vi "Grid_Read Control.vi"(8 "error in (no error)":errorcluster, 11 "Grid in":refnum<class "Grid.lvclass">) -> (0 "error out":errorcluster, 2 "Control":T1, 3 "Grid out":refnum<class "Grid.lvclass">)   [LabVIEW 2015, in "Grid.lvclass"]
uses:
  Grid.lvclass
  Grid_Control.ctl
  Grid.lvclass/Grid.ctl
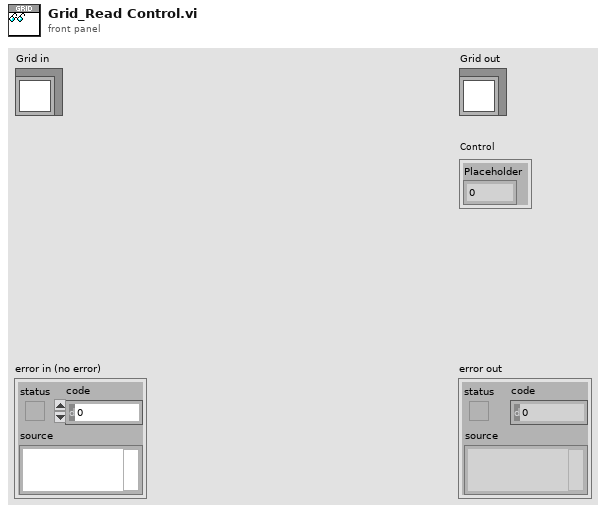
[diagram p1: front panel]
types:
  T1 = typedef "Grid.lvclass/Grid_Control.ctl" = cluster{"Placeholder":dbl}
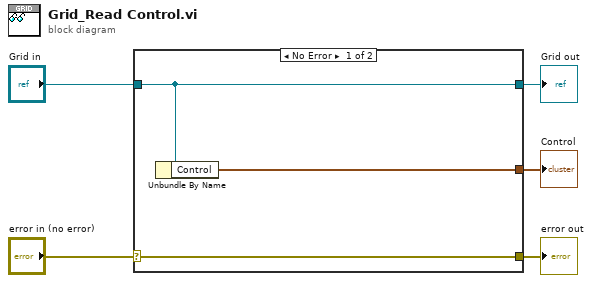
[diagram p0: block diagram]
diagram:
  n1 = case shown="No Error" "error in (no error)" {
    selector: "error in (no error)" -> [w8 w9]
    tunnel: [w8 w9] -> w4
    tunnel: [w7 w10] -> w2
    tunnel: "Grid in" -> [w7 w10]
    tunnel: [w6 _] -> w1
    frame No Error {
      n2 = Unbundle By Name(w7) -> ("Control"=w6:T1)
    }
    frame Error {
    }
  }
  "error out" <- w4
  "Grid out" <- w2
  "Control" <- w1
